vi "Resample N Waveforms (continuous).vi"(0 "waveforms in":waveform(dbl)[](array[waveform]), 1 "reset":bool, 5 "dt":dbl=1.0 format="%.2p", 7 "t0":timestamp=timestamp(-9223372036854775808 s since 1904-01-01) format="%<%.4X>T", 9 "interpolation mode":u16(ring)=1 items=["coerce", "linear", "spline", "FIR filter"], 11 "error in (no error)":errorcluster, 12 "FIR filter specifications":T1={"alias rejection (dB)"=120.0, "normalized bandwidth"=0.4536} {"normalized bandwidth" format="%.4f"; "alias rejection (dB)" format="%.2f"}) -> (4 "resampled waveforms out":waveform(dbl)[](array[waveform]), 8 "next t0's":timestamp[](array[timestamp]) format="%<%.4X>T", 10 "used t0's":timestamp[](array[timestamp]) format="%<%.4X>T", 14 "t0 adjusted warnings":bool[](array[boolean]), 15 "error out":errorcluster)   [LabVIEW 2020, in "NI_MAPro.lvlib"]
doc: "Resamples an input waveform according to the user-defined values for <B>t0</B> and <B>dt</B>. Wire data to the <B>waveform in</B> input to determine the polymorphic instance to use or manually select the instance."
uses:
  NI_MAPro.lvlib
  NI_MABase.lvlib
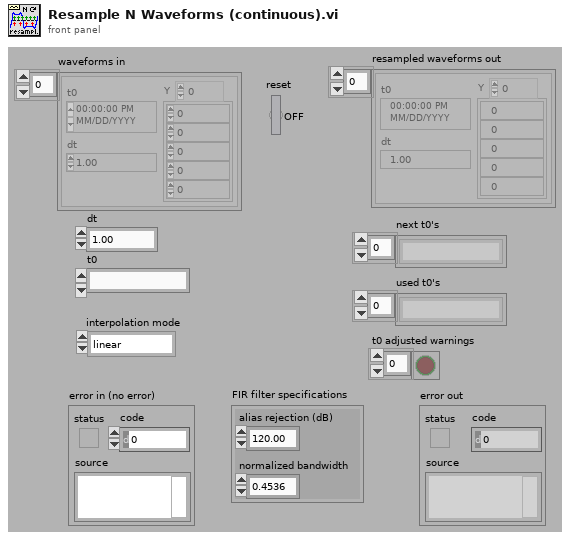
[diagram p1: front panel]
types:
  T1 = cluster{"alias rejection (dB)":dbl, "normalized bandwidth":dbl}
  T2 = cluster{"scaled filter":dbl[], "sub-filter size":i32, "filter max index":i32, "FIR index step":dbl, "half duration":dbl}
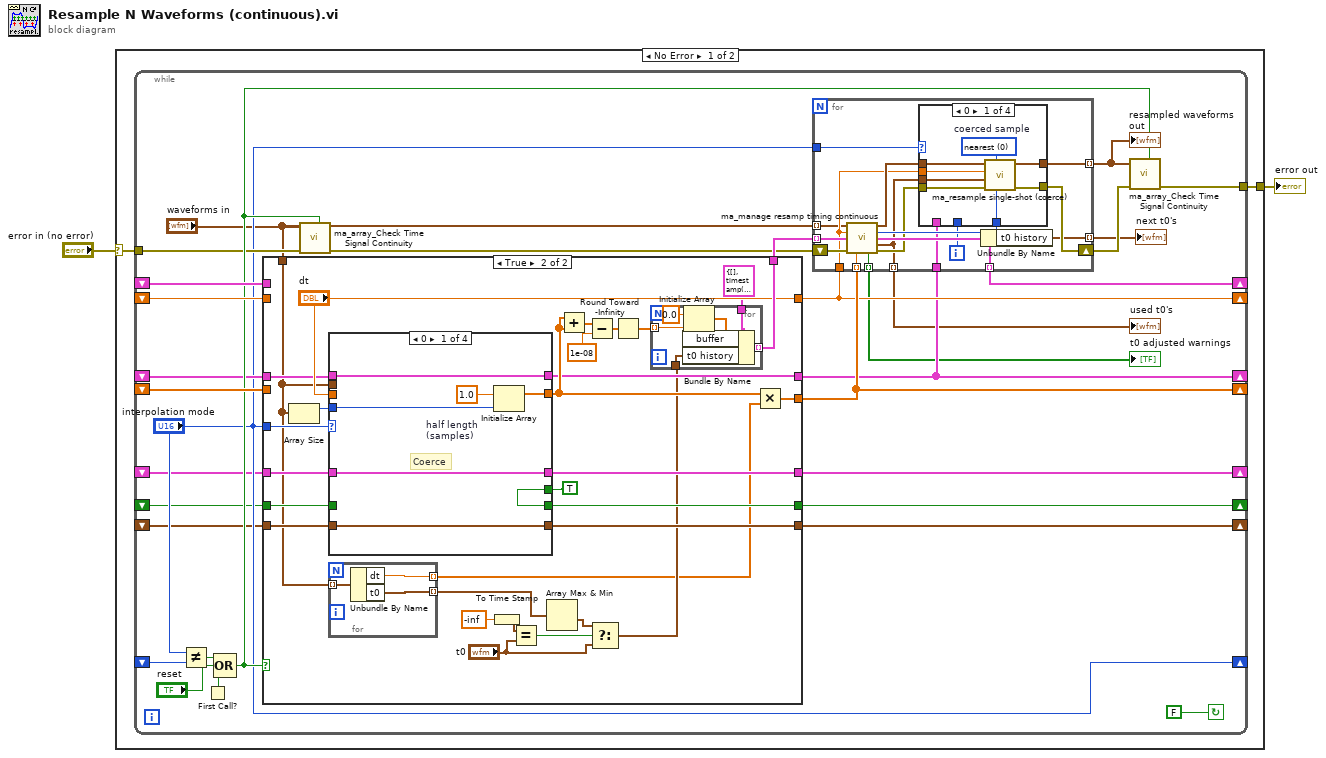
[diagram p0: block diagram]
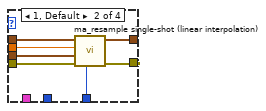
[diagram p2: hidden frame]
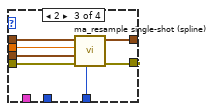
[diagram p3: hidden frame]
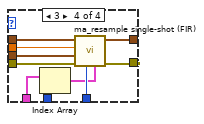
[diagram p4: hidden frame]
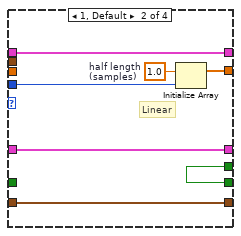
[diagram p6: hidden frame]
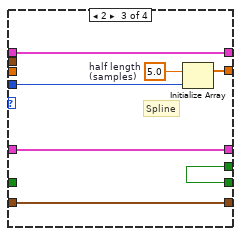
[diagram p7: hidden frame]
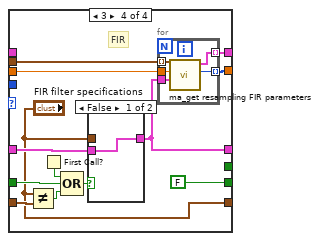
[diagram p8: hidden frame]
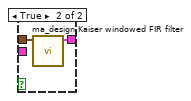
[diagram p9: hidden frame]
diagram:
  n1 = case shown="No Error" "error in (no error)" {
    selector: "error in (no error)" -> [w3 w172]
    tunnel: [w4 w172] -> w2
    frame No Error {
      n2 = while {
        shift-right: [w30] -> _
        shift-left: _ -> [w33]
        shift-right: ["interpolation mode"] -> _
        shift-left: _ -> [w17]
        shift-right: [w32] -> _
        shift-left: _ -> [w31]
        shift-right: [w26] -> _
        shift-left: _ -> [w29]
        shift-right: [w25] -> _
        shift-left: _ -> [w24]
        tunnel: [w23] -> w4
        tunnel: w3 -> [w22]
        shift-right: [w13] -> _
        shift-left: _ -> [w11]
        shift-right: [w12] -> _
        shift-left: _ -> [w10]
        shift-right: [w9] -> _
        shift-left: _ -> [w8]
        stop <- FALSE continue-if-true
        n3 = Not Equal?(x="interpolation mode", y=w17) -> (x != y?=w15:bool)
        n4 = First Call?() -> (First Call?: T/F=w16:bool)
        n5 = Compound Arithmetic op=OR(w15, "reset", w16) -> (w27:bool)
        n6 = case shown="True" w27 {
          tunnel: [w90 w120] -> w32
          tunnel: "interpolation mode" -> [_ w110]
          tunnel: [w91 w115] -> w34
          tunnel: w33 -> [w91 _]
          tunnel: w31 -> [w90 _]
          tunnel: [w89 "dt"] -> w26
          tunnel: w29 -> [w89 _]
          tunnel: [w88 w113] -> w25
          tunnel: w24 -> [w88 w102]
          tunnel: "waveforms in" -> [_ w101]
          tunnel: [w86 w108] -> w13
          tunnel: [w85 w107] -> w12
          tunnel: w11 -> [w86 w106]
          tunnel: w10 -> [w85 w105]
          tunnel: [w87 w104] -> w9
          tunnel: w8 -> [w87 w103]
          frame False {
          }
          frame True {
            n7 = Array Size(array=w101) -> (size(s)=w109:i32)
            n8 = case shown="0" w110 {
              tunnel: [w126 w133 w139 w157] -> w114
              tunnel: [w130 w137 w141 w156] -> w113
              tunnel: w102 -> [w130 w137 w141 _]
              tunnel: w101 -> [_ _ _ w155]
              tunnel: "dt" -> [_ _ _ w154]
              tunnel: [w129 w136 w144 w153] -> w104
              tunnel: w103 -> [w129 w136 w144 w152]
              tunnel: [w128 w135 w143 FALSE] -> w108
              tunnel: w106 -> [_ _ _ w148]
              tunnel: TRUE -> [w128 w135 w143 _]
              tunnel: [w127 w134 w142 "FIR filter specifications"] -> w107
              tunnel: w105 -> [w127 w134 w142 w150]
              tunnel: w109 -> [w124 w131 w138 _]
              frame 0 {
                w125 = 1.0  # half length (samples)
                # "Coerce"
                n9 = Initialize Array(w125, w124) -> (w126:dbl[])
              }
              frame 1, Default {
                w132 = 1.0  # half length (samples)
                # "Linear"
                n10 = Initialize Array(w132, w131) -> (w133:dbl[])
              }
              frame 2 {
                w140 = 5.0  # half length (samples)
                # "Spline"
                n11 = Initialize Array(w140, w138) -> (w139:dbl[])
              }
              frame 3 {
                # "FIR"
                n12 = Not Equal?(x="FIR filter specifications", y=w150) -> (x != y?=w149:bool)
                n13 = First Call?() -> (First Call?: T/F=w146:bool)
                n14 = Compound Arithmetic op=OR(w146, w148, w149) -> (w151:bool)
                n15 = case shown="False" w151 {
                  tunnel: [w163 w165] -> w153
                  tunnel: "FIR filter specifications" -> [_ w164]
                  tunnel: w152 -> [w163 _]
                  frame False {
                  }
                  frame True {
                    n16 = call "ma_design Kaiser windowed FIR filter.vi"("FIR filter specifications"=w164) -> ("filter data"=w165:cluster{"h":dbl[], "Max Decimation":dbl})  [unwired: 8 in, 1 out]
                  }
                }
                n17 = for {
                  tunnel: [w162] -> w157 mode=indexing
                  tunnel: [w161] -> w156 mode=indexing
                  tunnel: w155 -> [w160] mode=indexing
                  tunnel: w154 -> [w159]
                  tunnel: w153 -> [w158]
                  n18 = call "ma_get resampling FIR parameters.vi"("filter info"=w158, "dt"=w159, "Waveform in"=w160) -> ("history size"=w162:i32, "Filter parameters"=w161:T2)  [unwired: 7 in]
                }
              }
            }
            n19 = for {
              tunnel: w101 -> [w123] mode=indexing
              tunnel: [w121] -> w100 mode=indexing
              tunnel: [w122] -> w97 mode=indexing
              n20 = Unbundle By Name(w123) -> ("dt"=w122:dbl, "t0"=w121:timestamp)
            }
            n21 = To Time Stamp(1:-inf ("x")) -> (0:w94:timestamp)
            n22 = Equal?(x=w94, y="t0") -> (x = y?=w93:bool)
            n23 = Array Max & Min(array=w100) -> (min value=w99:timestamp)  [unwired: 3 out]
            n24 = Add(x=w114, y=w114) -> (x+y=w119:dbl[])
            n25 = Subtract(x=w119, y=1e-08) -> (x-y=w117:dbl[])
            n26 = Select(t=w99, s=w93, f="t0") -> (s? t:f=w98:timestamp)
            n27 = Round Toward -Infinity(1:w117) -> (0:w116:dbl[])
            n28 = for {
              tunnel: w116 -> [w168] mode=indexing
              tunnel: [w167] -> w115 mode=indexing
              tunnel: w98 -> [w169]
              tunnel: cluster{"buffer":dbl[], "t0 history":timestamp} {"buffer"=[], "t0 history"=timestamp(0 s since 1904-01-01)} ("state info in") -> [w166]
              n29 = Initialize Array(0.0 ("element"), w168) -> (w170:dbl[])
              n30 = Bundle By Name(cluster=w166, "buffer"=w170, "t0 history"=w169) -> (w167:cluster{"buffer":dbl[], "t0 history":timestamp})
            }
            n31 = Multiply(x=w114, y=w97) -> (x*y=w120:dbl[])
          }
        }
        n32 = call "ma_array_Check Time Signal Continuity.vi"("Ignore input time stamp"=w27, "error in (no error)"=w22, "waveforms"="waveforms in") -> ("error out"=w21:errorcluster)  [unwired: 5 in, 3 out]
        n33 = for {
          tunnel: w34 -> [w51] mode=indexing
          tunnel: w32 -> [w50] mode=indexing
          tunnel: [w49] -> w30 mode=indexing
          tunnel: "interpolation mode" -> [w48]
          tunnel: [w44] -> w14 mode=indexing
          tunnel: w26 -> [w43]
          tunnel: w25 -> [w36]
          tunnel: "waveforms in" -> [w42] mode=indexing
          shift-right: [w41] -> w20
          shift-left: w21 -> [w52]
          tunnel: [w40] -> w6 mode=indexing
          tunnel: [w39] -> w19 mode=indexing
          tunnel: [w38] -> w5 mode=indexing
          i -> [w37]
          n34 = call "ma_manage resamp timing continuous.vi"("waveform in"=w42, "dt"=w43, "state info in"=w51, "error in"=w52, "filter half-length (s)"=w50) -> ("waveform to be processed"=w47:waveform(dbl), "#elements"=w46:i32, "state info out"=w49:cluster{"buffer":dbl[], "t0 history":timestamp}, "used t0"=w40:timestamp, "t0 adjusted warning"=w39:bool, "error out"=w45:errorcluster)  [unwired: 5 in]
          n35 = case shown="0" w48 {
            tunnel: w47 -> [w60 w67 w74 w84]
            tunnel: w46 -> [w53 w61 w68 w78]
            tunnel: w40 -> [w59 w66 w73 w83]
            tunnel: w43 -> [w58 w65 w72 w82]
            tunnel: w45 -> [w57 w64 w71 w81]
            tunnel: [w56 w63 w70 w80] -> w41
            tunnel: [w55 w62 w69 w79] -> w44
            tunnel: w37 -> [_ _ _ w76]
            tunnel: w36 -> [_ _ _ w75]
            frame 0 {
              w54 = u16 0 items=["nearest", "previous", "next"]  # coerced sample
              n36 = call "ma_resample single-shot (coerce).vi"("#elements"=w53, "coerced sample"=w54, "error in"=w57, "t0"=w59, "dt"=w58, "waveform in"=w60) -> ("error out"=w56:errorcluster, "resampled waveform out"=w55:waveform(dbl))  [unwired: 4 in]
            }
            frame 1, Default {
              n37 = call "ma_resample single-shot (linear interpolation).vi"("#elements"=w61, "error in"=w64, "t0"=w66, "dt"=w65, "waveform in"=w67) -> ("error out"=w63:errorcluster, "resampled waveform out"=w62:waveform(dbl))  [unwired: 5 in]
            }
            frame 2 {
              n38 = call "ma_resample single-shot (spline).vi"("#elements"=w68, "error in"=w71, "t0"=w73, "dt"=w72, "waveform in"=w74) -> ("error out"=w70:errorcluster, "resampled waveform out"=w69:waveform(dbl))  [unwired: 3 in, 2 out]
            }
            frame 3 {
              n39 = Index Array(array=w75, index=w76) -> (element=w77:T2)
              n40 = call "ma_resample single-shot (FIR).vi"("Filter parameters"=w77, "#elements"=w78, "error in"=w81, "t0"=w83, "dt"=w82, "waveform in"=w84) -> ("error out"=w80:errorcluster, "resampled waveform out"=w79:waveform(dbl))  [unwired: 4 in]
            }
          }
          n41 = Unbundle By Name(w49) -> ("t0 history"=w38:timestamp)
        }
        "t0 adjusted warnings" <- w19
        "used t0's" <- w6
        "next t0's" <- w5
        "resampled waveforms out" <- w14
        n42 = call "ma_array_Check Time Signal Continuity.vi"("Ignore input time stamp"=w27, "error in (no error)"=w20, "waveforms"=w14) -> ("error out"=w23:errorcluster)  [unwired: 5 in, 3 out]
      }
    }
    frame Error {
    }
  }
  "error out" <- w2
